vi "Host_side_DAQ_data - Copy.vi"() -> ()   [LabVIEW 2017]
uses:
  <vilib>/Waveform/WDTOps.llb/WDT Append Waveforms DBL.vi
panel:
  out "Waveform Chart 3":waveform(dbl)(graph)
  out "Difference between signals 1 & 2":dbl
  out "Numeric 2":dbl
  out "Numeric":dbl
  out "Waveform Chart 2":waveform(dbl)(graph)
  in  "stop":bool
  out "Waveform Chart":waveform(dbl)(graph)
  in  "Recording Data":bool
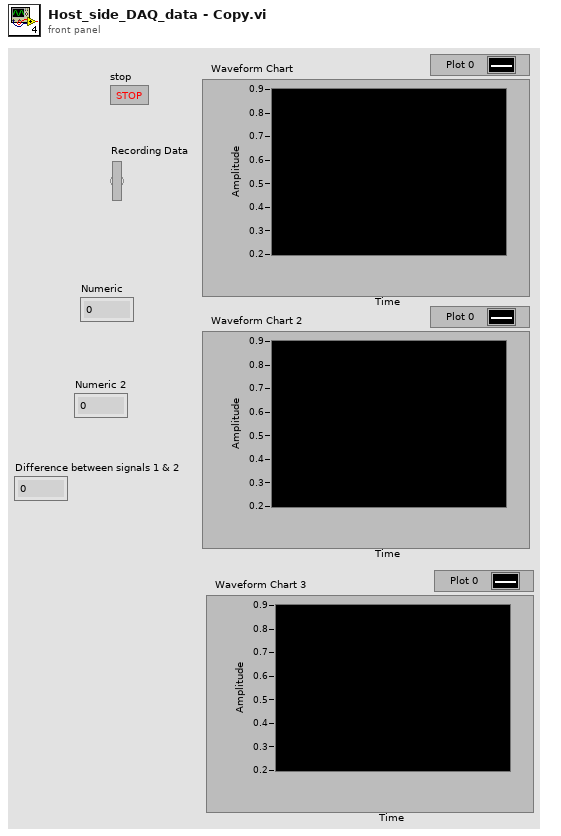
[diagram p1: front panel]
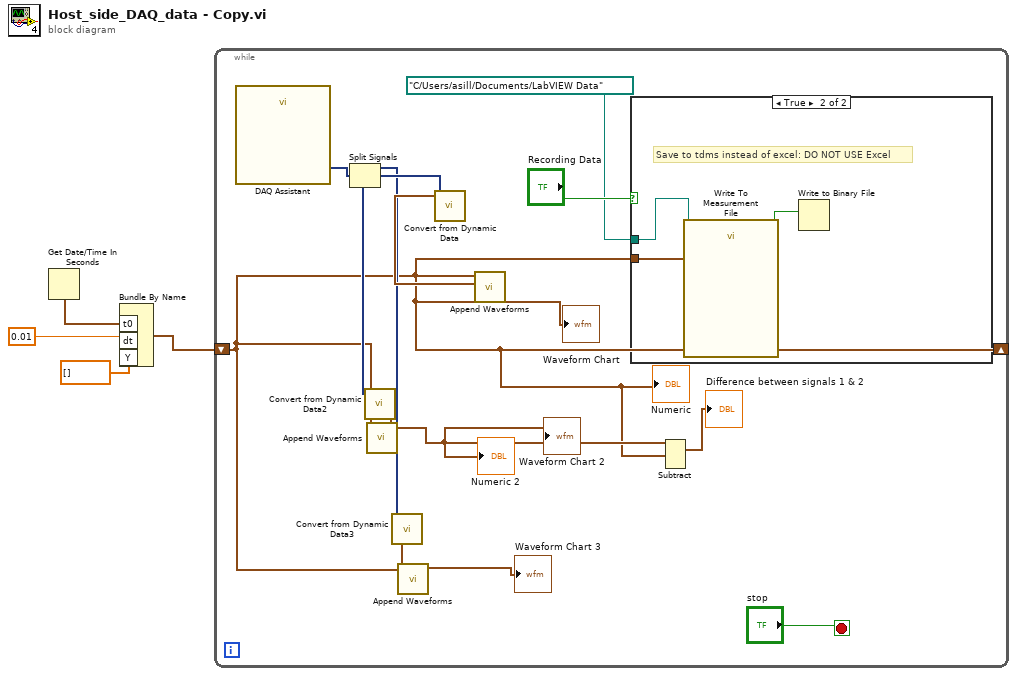
[diagram p0: block diagram]
diagram:
  n1 = Get Date/Time In Seconds() -> (seconds since 1Jan1904=w2:timestamp)
  n2 = Bundle By Name("t0"=w2, "dt"=0.01, "Y"=dbl[] []) -> (w3:waveform(dbl))  [unwired: 1 in]
  n3 = while {
    shift-right: [w10] -> _
    shift-left: w3 -> [w6]
    stop <- "stop" stop-if-true
    n4 = call "DAQ Assistant"() -> ("data"=w14:dynamicdata)  [unwired: 16 in, 3 out]
    n5 = Split Signals(w14) -> (w8:dynamicdata, w13:dynamicdata, w12:dynamicdata)  [unwired: 3 in]
    n6 = call "Convert from Dynamic Data2"("Dynamic Data Type"=w12) -> ("Waveform"=w15:waveform(dbl))  [unwired: 3 in]
    n7 = call-poly <vilib>:"Append Waveforms.vi"("waveform B"=w15, "waveform A"=w6) -> ("waveform out"=w11:waveform(dbl))  [unwired: 8 in, 1 out]
    "Waveform Chart 2" <- w11
    "Numeric 2" <- w11
    n8 = call "Convert from Dynamic Data3"("Dynamic Data Type"=w8) -> ("Waveform"=w7:waveform(dbl))  [unwired: 3 in]
    n9 = call-poly <vilib>:"Append Waveforms.vi"("waveform B"=w7, "waveform A"=w6) -> ("waveform out"=→"Waveform Chart 3":waveform(dbl))  [unwired: 8 in, 1 out]
    n10 = call "Convert from Dynamic Data"("Dynamic Data Type"=w13) -> ("Waveform"=w18:waveform(dbl))  [unwired: 3 in]
    n11 = call-poly <vilib>:"Append Waveforms.vi"("waveform B"=w18, "waveform A"=w6) -> ("waveform out"=w10:waveform(dbl))  [unwired: 8 in, 1 out]
    "Waveform Chart" <- w10
    "Numeric" <- w10
    n12 = case shown="True" "Recording Data" {
      tunnel: path "C:/Users/asill/Documents/LabVIEW Data" -> [_ w21]
      tunnel: w10 -> [_ w20]
      frame False {
      }
      frame True {
        # "Save to tdms instead of excel: DO NOT USE Excel"
        n13 = call "Write To Measurement File"("Signals"=w20, "Filename"=w21) -> ("Saving Data"=w22:bool)  [unwired: 15 in, 2 out]
        n14 = Write to Binary File(data=w22) -> ()  [unwired: 5 in, 3 out]
      }
    }
    n15 = Subtract(1:w10, 2:w11) -> (0:→"Difference between signals 1 & 2":waveform(dbl))  [unwired: 1 in, 1 out]
  }
